vi "GenericStatusIndicator.vi"(9 "Total":i32, 10 "Current Iteration":i32, 11 "String in":refnum<vi>) -> (3 "Status":string)   [LabVIEW 2023, in "Reusables.lvlib"]
uses:
  Reusables.lvlib
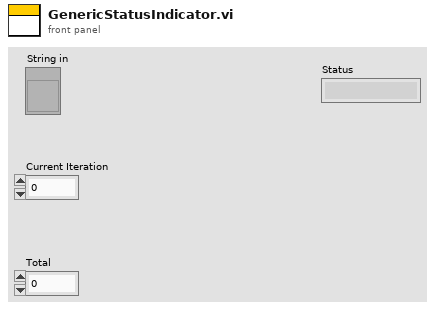
[diagram p1: front panel]
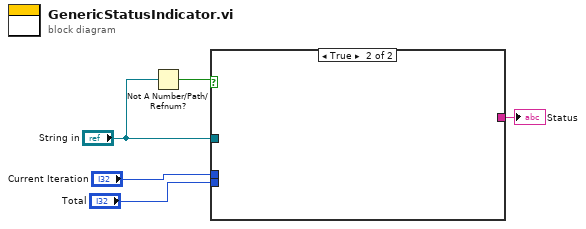
[diagram p0: block diagram]
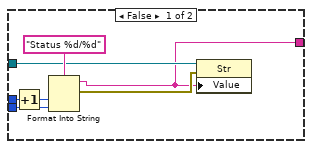
[diagram p2: hidden frame]
diagram:
  n1 = Not A Number/Path/Refnum?(number/path/refnum="String in") -> (NaN/Path/Refnum?=w2:bool)
  n2 = case shown="True" w2 {
    tunnel: "Current Iteration" -> [w11 _]
    tunnel: "Total" -> [w10 _]
    tunnel: "String in" -> [w8 _]
    tunnel: [w6 _] -> w1
    frame False {
      n3 = Increment(x=w11) -> (x+1=w7:i32)
      n4 = Format Into String(format string="Status %d/%d", w7, w10) -> (resulting string=w6:string, error out=w12:errorcluster)  [unwired: 2 in]
      n5 = property class="Str"(reference=w8, error in=w12, "Value"=w6) -> ()  [unwired: 2 out]
    }
    frame True {
    }
  }
  "Status" <- w1
